vi "Signal_Create.vi"(0 "reference in":refnum<class "Signal.lvclass">, 5 "error in (no error)":errorcluster) -> (14 "reference out":refnum<class "Signal.lvclass">, 19 "error out":errorcluster)   [LabVIEW 2019]
doc: "Constructor."
uses:
  <vilib>/addons/_AddQ/G#Object/G#Object.lvclass
  Signal.lvclass
  D:/LabASF/LabASF/src/Proccess_class/Proccess.lvclass
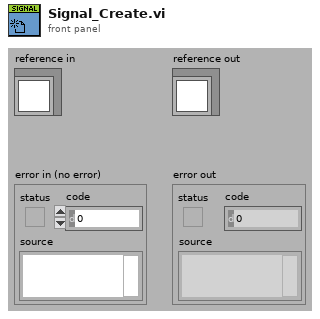
[diagram p1: front panel]
types:
  T1 = typedef "Signal.lvclass/ObjectAttributesRef.ctl" = refnum<data-value>
  T2 = typedef "Signal.lvclass/ObjectAttributes.ctl" = cluster{"Alarm":bool, "Warning":bool, "ForceMode":bool}
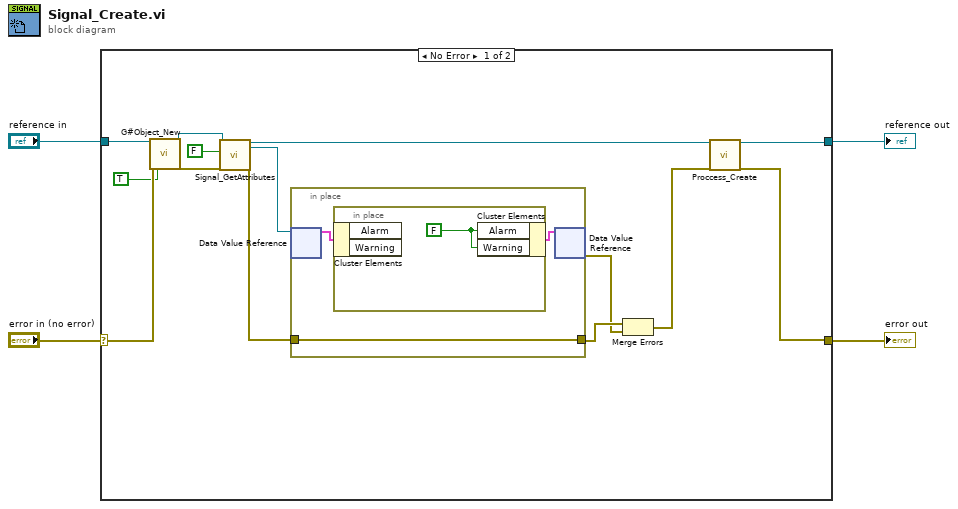
[diagram p0: block diagram]
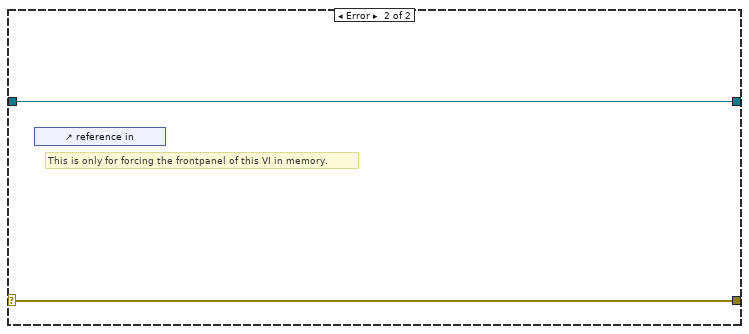
[diagram p2: hidden frame]
diagram:
  n1 = case shown="No Error" "error in (no error)" {
    selector: "error in (no error)" -> [w17 w24]
    tunnel: [w5 w24] -> w3
    tunnel: [w7 w23] -> w1
    tunnel: "reference in" -> [w18 w23]
    frame No Error {
      n2 = call <vilib>:"G#Object_New.vi"("reference in"=w18, "error in (no error)"=w17, "user counter (T)?"=TRUE ("User Counter")) -> ("reference out"=w10:refnum<class "G#Object.lvclass">, "error out"=w9:errorcluster)  [unwired: 14 in, 1 out]
      n3 = call "Signal_GetAttributes.vi"("reference in"=w10, "return data? (T)"=FALSE ("return data"), "error in (no error)"=w9) -> ("reference out"=w8:refnum<class "Signal.lvclass">, "attributes ref"=w12:T1, "error out"=w13:errorcluster)  [unwired: 13 in, 1 out]
      n4 = in-place {
        in-place-border: w13 -> [w19]
        in-place-border: [w19] -> w15
        n5 = in-place-dvr #1(w12) -> (w20:T2)  [unwired: 1 out]
        n6 = in-place {
          w22 = FALSE ("Alarm")
          n7 = in-place-cluster #2(w20) -> ()  [unwired: 2 out]
          n8 = in-place-cluster #2("Alarm"=w22, "Warning"=w22) -> (w21:T2)
        }
        n9 = in-place-dvr #1(w21) -> (w14:errorcluster)  [unwired: 1 out]
      }
      n10 = Merge Errors(w15, w14) -> (w6:errorcluster)
      n11 = call "Proccess_Create.vi"("reference in"=w8, "error in (no error)"=w6) -> ("reference out"=w7:refnum<class "Signal.lvclass">, "error out"=w5:errorcluster)  [unwired: 16 in]
    }
    frame Error {
      # "This is only for forcing the frontpanel of this VI in memory."
      n12 = control-ref of="reference in"() -> ()  [unwired: 1 out]
    }
  }
  "error out" <- w3
  "reference out" <- w1
